vi "OFDM RX_syh.vi"() -> ()   [LabVIEW 2013]
uses:
  <vilib>/addons/Modulation/Analog/controls/Complex Data Waveform.ctl
  <vilib>/Analysis/2dsp.llb/Complex FFT.vi
  <vilib>/addons/Modulation/Digital/General/MT Map QAM Symbols to Bits.vi
  <vilib>/addons/Modulation/niAMT.lvlib
  <vilib>/Analysis/NI_AALPro.lvlib
  <vilib>/addons/Modulation/niDMT.lvlib
panel:
  out "Complex baseband":cluster{"t0":dbl, "dt":dbl, "Y":dbl[]}[](graph)
  out "Constellation":cdb[](graph)
  out "Bit Error Rate":dbl
  out "output cluster":cluster{bool[], bool[]}
  out "error out":errorcluster
  in  "error in (no error)":errorcluster
  in  "desired sample rate (Hz)":dbl=1.0 format="%.2f"
  in  "Queue size":i32
  in  "stop":bool
  # "OFDM Receiver"
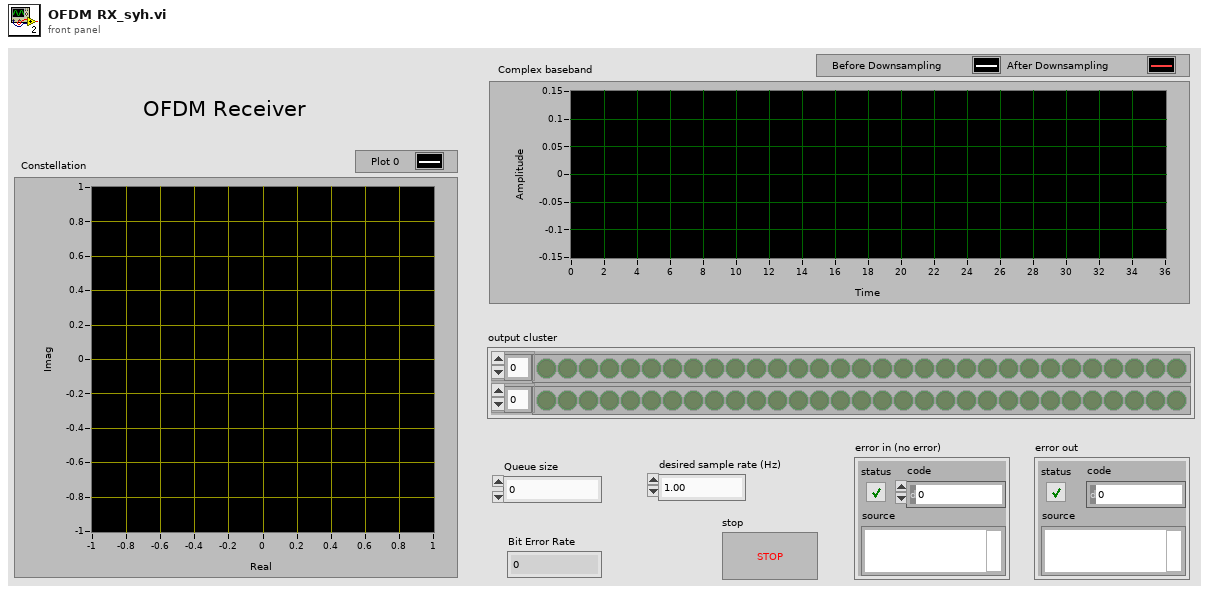
[diagram p1: front panel]
types:
  T1 = cluster{"IQ Data":cdb[], "Original Bitstream":i8[]}
  T2 = typedef "niAMT.lvlib/Complex Data Waveform.ctl" = cluster{"t0":dbl, "dt":dbl, "Y":cdb[]}
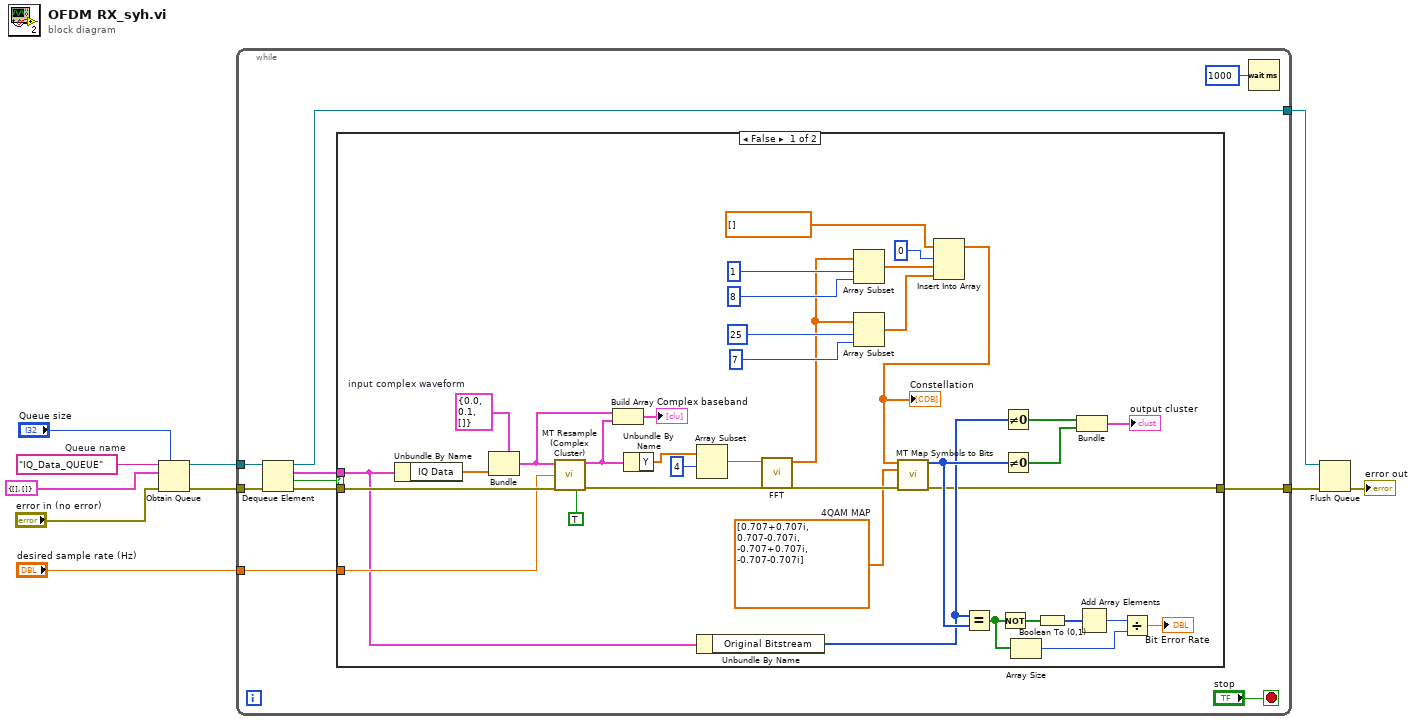
[diagram p0: block diagram]
diagram:
  w10 = "IQ_Data_QUEUE"  # Queue name
  n1 = Obtain Queue(max queue size (-1, unlimited)="Queue size", name (unnamed)=w10, element data type=T1 {"IQ Data"=[], "Original Bitstream"=[]}, error in (no error)="error in (no error)") -> (queue out=w6:refnum<queue>, error out=w5:errorcluster)  [unwired: 1 in, 1 out]
  n2 = while {
    tunnel: w6 -> [w18]
    tunnel: w5 -> [w17]
    tunnel: [w15] -> w4
    tunnel: [w13] -> w2
    tunnel: "desired sample rate (Hz)" -> [w11]
    stop <- "stop" stop-if-true
    n3 = Dequeue Element(queue=w18, error in (no error)=w17) -> (queue out=w13:refnum<queue>, element=w12:T1, timed out?=w16:bool, error out=w14:errorcluster)  [unwired: 1 in]
    n4 = case shown="False" w16 {
      tunnel: [w35 w57] -> w15
      tunnel: w14 -> [w53 w57]
      tunnel: w12 -> [w47 _]
      tunnel: w11 -> [w49 _]
      frame False {
        w55 = T2 {"t0"=0.0, "dt"=0.1, "Y"=[]}  # input complex waveform
        w48 = cdb[] [0.707+0.707i, 0.707-0.707i, -0.707+0.707i, -0.707-0.707i]  # 4QAM MAP
        n5 = Unbundle By Name(w47) -> ("IQ Data"=w56:cdb[])
        n6 = Bundle(cluster=w55, "Y"=w56) -> (w50:T2)  [unwired: 2 in]
        n7 = call <vilib>:"MT Resample (Complex Cluster).vi"("input complex waveform"=w50, "desired sample rate (Hz)"=w49, "error in (no error)"=w53, "flush buffers? (F)"=TRUE) -> ("output complex waveform"=w51:T2, "error out"=w52:errorcluster)  [unwired: 10 in]
        n8 = Build Array(w50, w51) -> (→"Complex baseband":T2[])
        n9 = Unbundle By Name(w51) -> ("Y"=w32:cdb[])
        n10 = Array Subset(array=w32, index=4) -> (w31:cdb[])  [unwired: 1 in]
        n11 = Unbundle By Name(w47) -> ("Original Bitstream"=w41:i8[])
        n12 = call-poly <vilib>:"FFT.vi"("X"=w31) -> ("FFT {X}"=w26:cdb[])  [unwired: 9 in, 1 out]
        n13 = Array Subset(array=w26, index=1, length=8) -> (w24:cdb[])
        n14 = Array Subset(array=w26, index=25, length=7) -> (w22:cdb[])
        n15 = Insert Into Array(array=cdb[] [], index=0, new element #1=w24, new element #2=w22) -> (w21:cdb[])
        "Constellation" <- w21
        n16 = call-poly <vilib>:"MT Map Symbols to Bits.vi"("symbols"=w21, "symbol map"=w48, "error in (no error)"=w52) -> ("output bit stream"=w42:i8[], "error out"=w35:errorcluster)  [unwired: 11 in]
        n17 = Equal?(x=w41, y=w42) -> (x = y?=w40:bool[])
        n18 = Not(x=w40) -> (.not. x?=w39:bool[])
        n19 = Not Equal To 0?(x=w41) -> (x != 0?=w45:bool[])
        n20 = Not Equal To 0?(x=w42) -> (x != 0?=w44:bool[])
        n21 = Array Size(array=w40) -> (size(s)=w37:i32)
        n22 = Boolean To (0,1)(Boolean=w39) -> (0, 1=w38:i16[])
        n23 = Bundle(w45, w44) -> (→"output cluster":cluster{bool[], bool[]})  [unwired: 1 in]
        n24 = Add Array Elements(numeric array=w38) -> (sum=w46:i16)
        n25 = Divide(x=w46, y=w37) -> (x/y=→"Bit Error Rate":dbl)
      }
      frame True {
      }
    }
    n26 = Wait (ms)(milliseconds to wait=u32 1000) -> ()  [unwired: 1 out]
  }
  n27 = Flush Queue(queue=w2, error in (no error)=w4) -> (error out=→"error out":errorcluster)  [unwired: 2 out]
